vi "Untitled 1 (SubVI).vi"(0 "Byte Stream File in":refnum<file>, 1 "file open?":bool, 2 "CSV Data Headings":string, 3 "millisecond timer value in":u32, 4 "Start Logging":bool, 5 "error in (no error)":errorcluster, 6 "Log Filepath Selection":T2, 7 "adam5000:all-data-out":T3) -> (10 "appended path for log file":path, 12 "UI Element State":T1(ring), 13 "log-elapsed time":dbl format="%.2f", 14 "Byte Stream File out":refnum<file>, 15 "millisecond timer value out":u32, 16 "Logged Data String":string, 17 "Boolean":bool, 18 "Boolean 2":bool, 19 "error out":errorcluster)   [LabVIEW 2024]
uses:
  controls/thermocouple-input-cluster.ctl
  controls/analog-input-cluster.ctl
  controls/analog-output-cluster.ctl
  controls/digitial-input-cluster.ctl
  controls/digital-output-cluster.ctl
  controls/adam-5000-all-module-datas.ctl
  controls/adam-5000-all-chassis-data.ctl
  csv-file-logging/filepath-selection.ctl
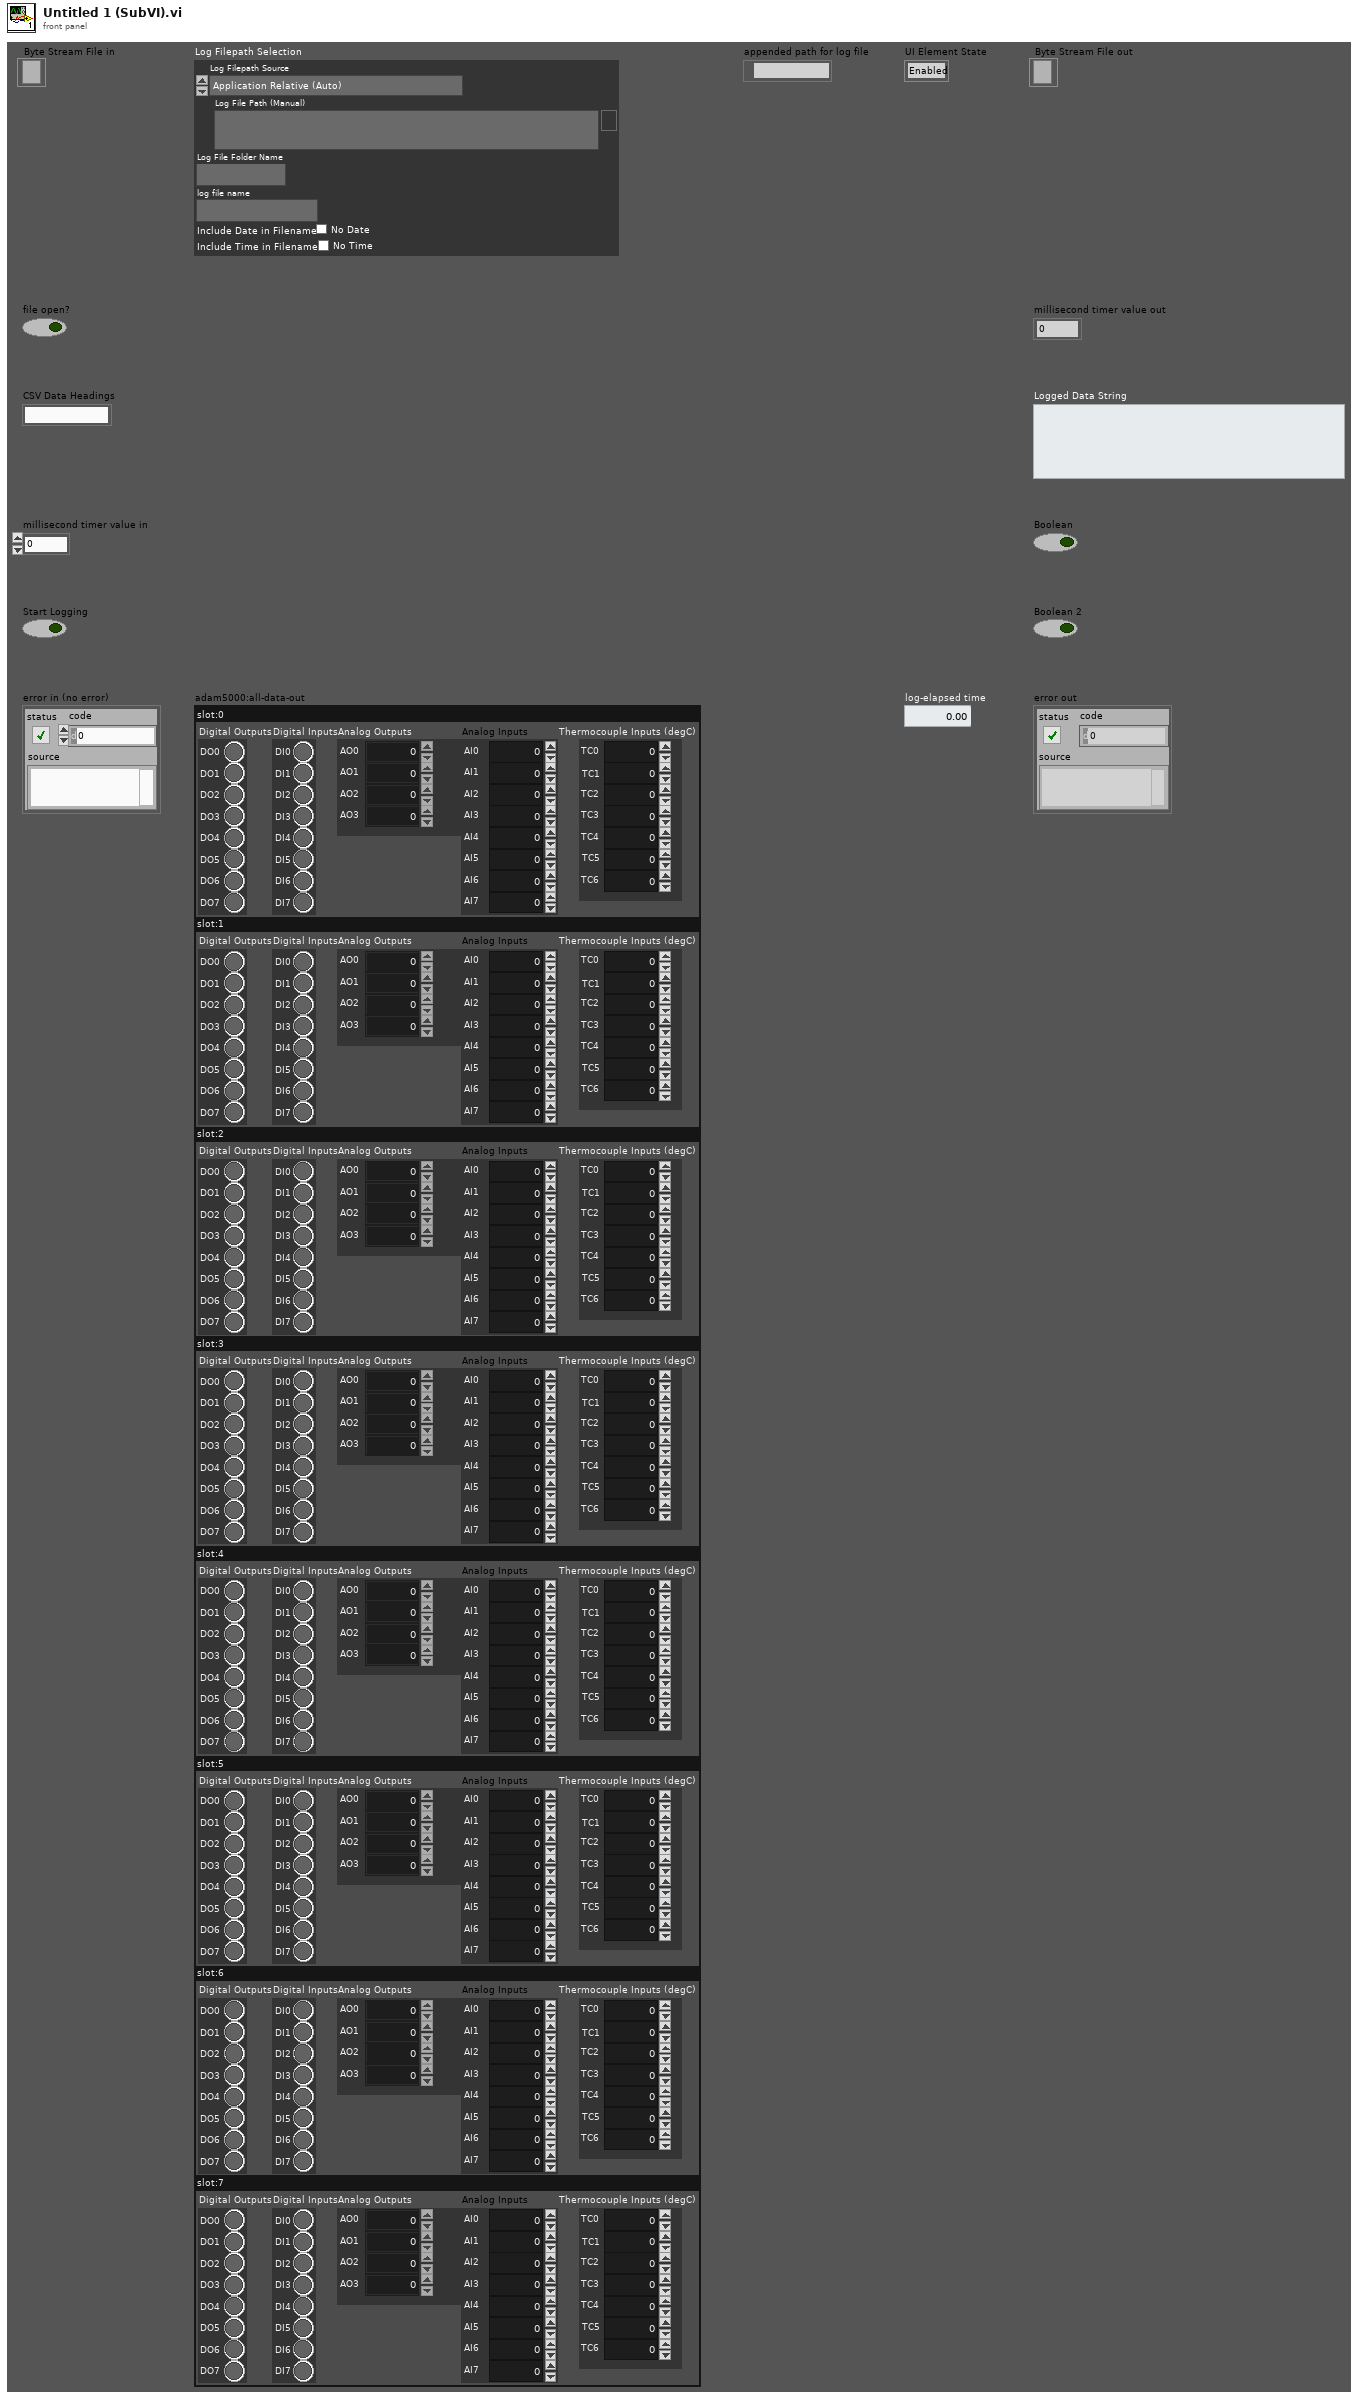
[diagram p1: front panel]
types:
  T1 = enum8{"Enabled", "Disabled", "Disabled and Grayed Out"}
  T2 = typedef "filepath-selection.ctl" = cluster{"Log Filepath Source":enum16{"Application Relative (Auto)", "VI Relative (Auto)", "Complete Path (Manual)"}, "Log File Path (Manual)":path, "Log File Folder Name":string, "log file name":string, "Include Date in Filename":bool, "Include Time in Filename":bool}
  T3 = typedef "adam-5000-all-chassis-data.ctl" = cluster{"slot:0":T4, "slot:1":T4, "slot:2":T4, "slot:3":T4, "slot:4":T4, "slot:5":T4, "slot:6":T4, "slot:7":T4}
  T4 = typedef "adam-5000-all-module-datas.ctl" = cluster{"Digital Outputs":T5, "Digital Inputs":T6, "Analog Outputs":T7, "Analog Inputs":T8, "Thermocouple Inputs (degC)":T9}
  T5 = typedef "digital-output-cluster.ctl" = cluster{"DO0":bool, "DO1":bool, "DO2":bool, "DO3":bool, "DO4":bool, "DO5":bool, "DO6":bool, "DO7":bool}
  T6 = typedef "digitial-input-cluster.ctl" = cluster{"DI0":bool, "DI1":bool, "DI2":bool, "DI3":bool, "DI4":bool, "DI5":bool, "DI6":bool, "DI7":bool}
  T7 = typedef "analog-output-cluster.ctl" = cluster{"AO0":dbl, "AO1":dbl, "AO2":dbl, "AO3":dbl}
  T8 = typedef "analog-input-cluster.ctl" = cluster{"AI0":dbl, "AI1":dbl, "AI2":dbl, "AI3":dbl, "AI4":dbl, "AI5":dbl, "AI6":dbl, "AI7":dbl}
  T9 = typedef "thermocouple-input-cluster.ctl" = cluster{"TC0":dbl, "TC1":dbl, "TC2":dbl, "TC3":dbl, "TC4":dbl, "TC5":dbl, "TC6":dbl}
  T10 = enum16{"open", "replace", "create", "open or create", "replace or create", "replace or create with confirmation"}
  T11 = cluster{"TC0":string, "TC1":string, "TC2":string, "TC3":string, "TC4":string, "TC5":string, "TC6":string}
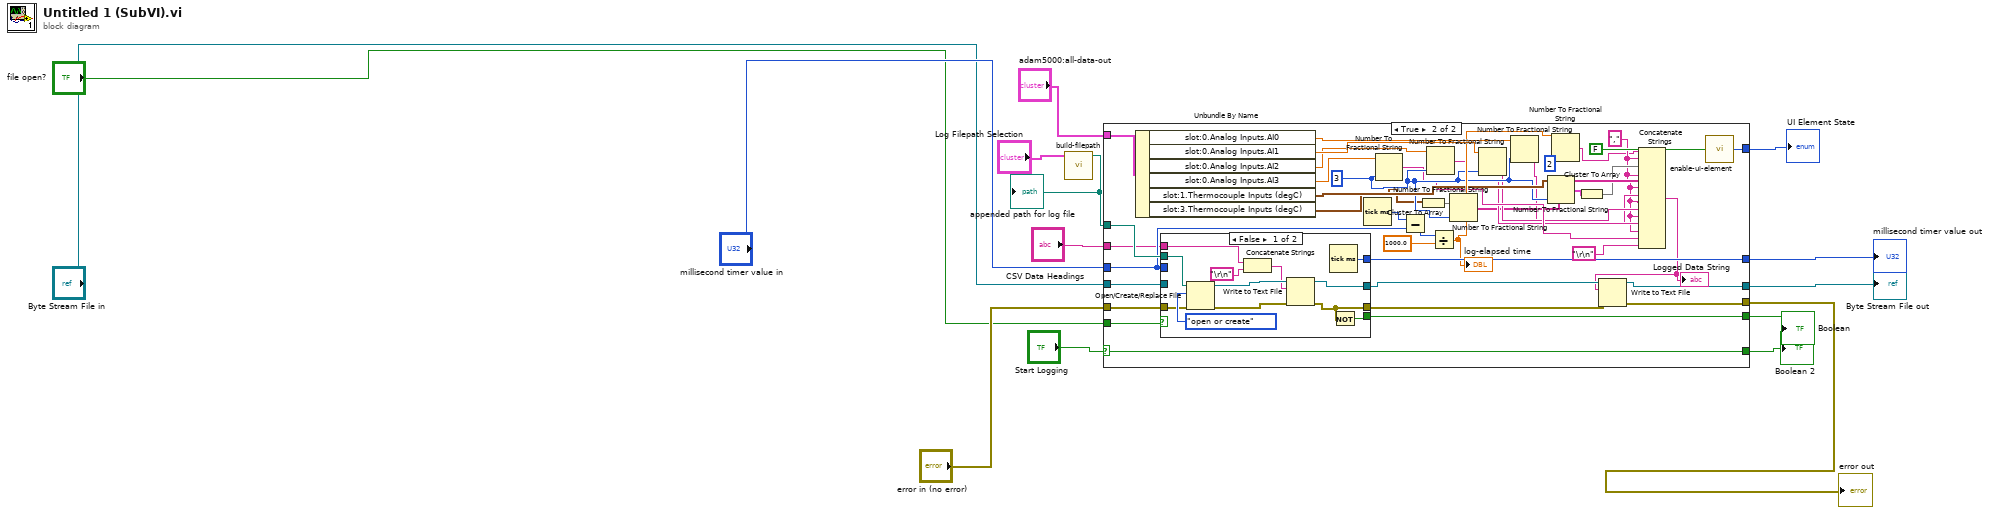
[diagram p0: block diagram]
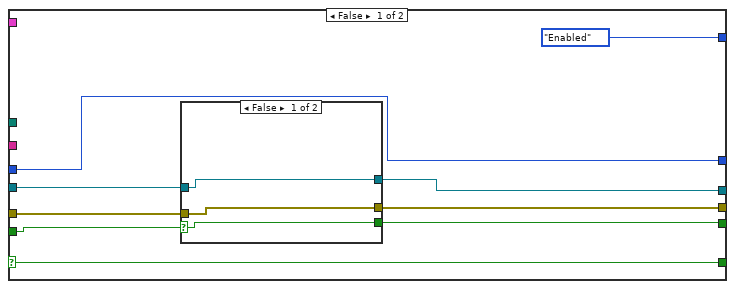
[diagram p2: hidden frame]
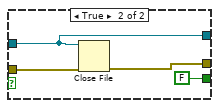
[diagram p3: hidden frame]
diagram:
  n1 = call "build-filepath.vi"("Log Filepath Selection"="Log Filepath Selection") -> ("appended path for log file"=w5:path)  [unwired: 9 in, 1 out]
  "appended path for log file" <- w5
  n2 = case shown="True" "Start Logging" {
    selector: "Start Logging" -> [w24 w68]
    tunnel: [w24 w68] -> w2
    tunnel: [T1."Enabled" ("DisabledEnum") w69] -> w3
    tunnel: w5 -> [_ w66]
    tunnel: "adam5000:all-data-out" -> [_ w71]
    tunnel: [w21 w64] -> w7
    tunnel: "file open?" -> [w22 w67]
    tunnel: "error in (no error)" -> [w19 w65]
    tunnel: [w18 w53] -> w10
    tunnel: [w17 w55] -> w11
    tunnel: "Byte Stream File in" -> [w20 w63]
    tunnel: [w16 w62] -> w13
    tunnel: "millisecond timer value in" -> [w16 w60]
    tunnel: "CSV Data Headings" -> [_ w57]
    frame False {
      n3 = case shown="False" w22 {
        selector: w22 -> [w25 _]
        tunnel: [w25 FALSE] -> w21
        tunnel: w20 -> [w27 w28]
        tunnel: w19 -> [w26 w30]
        tunnel: [w26 w29] -> w18
        tunnel: [w27 w28] -> w17
        frame False {
        }
        frame True {
          n4 = Close File(refnum=w28, error in=w30) -> (error out=w29:errorcluster)  [unwired: 1 out]
        }
      }
    }
    frame True {
      w33 = "," ("string")
      w44 = i16 3 ("precision (6)")
      n5 = Unbundle By Name(w71) -> ("slot:0.Analog Inputs.AI0"=w51:dbl, "slot:0.Analog Inputs.AI1"=w50:dbl, "slot:0.Analog Inputs.AI2"=w49:dbl, "slot:0.Analog Inputs.AI3"=w48:dbl, "slot:1.Thermocouple Inputs (degC)"=w45:T9, "slot:3.Thermocouple Inputs (degC)"=w41:T9)
      n6 = case shown="False" w67 {
        selector: w67 -> [_ w87]
        tunnel: w66 -> [w82 _]
        tunnel: w65 -> [w81 w86]
        tunnel: [w76 w86] -> w54
        tunnel: [w80 w87] -> w64
        tunnel: [w75 w84] -> w56
        tunnel: w63 -> [_ w84]
        tunnel: [w79 w85] -> w62
        tunnel: w60 -> [_ w85]
        tunnel: w57 -> [w73 _]
        frame False {
          n7 = Open/Create/Replace File(file path (use dialog)=w82, error in=w81, operation (0:open)=T10."open or create") -> (refnum out=w78:refnum<file>, error out=w77:errorcluster)  [unwired: 3 in, 1 out]
          n8 = Concatenate Strings(w73, "\r\n") -> (w72:string)
          n9 = Write to Text File(file (use dialog)=w78, text=w72, error in=w77) -> (refnum out=w75:refnum<file>, error out=w76:errorcluster)  [unwired: 1 in, 1 out]
          n10 = Tick Count (ms)() -> (millisecond timer value=w79:u32)
          n11 = Not(x=w76) -> (.not. x?=w80:bool)
        }
        frame True {
        }
      }
      n12 = Tick Count (ms)() -> (millisecond timer value=w61:u32)
      n13 = Number To Fractional String(number=w48, precision (6)=w44) -> (F-format string=w39:string)  [unwired: 2 in]
      n14 = Subtract(x=w61, y=w60) -> (x-y=w59:u32)
      n15 = Cluster To Array(cluster=w41) -> (array=w40:dbl[])
      n16 = Number To Fractional String(number=w49, precision (6)=w44) -> (F-format string=w38:string)  [unwired: 2 in]
      n17 = Divide(x=w59, y=1000.0) -> (x/y=w46:dbl)
      "log-elapsed time" <- w46
      n18 = Number To Fractional String(number=w40, precision (6)=w44) -> (F-format string=w35:string[])  [unwired: 2 in]
      n19 = Number To Fractional String(number=w50, precision (6)=w44) -> (F-format string=w37:string)  [unwired: 2 in]
      n20 = Number To Fractional String(number=w51, precision (6)=w44) -> (F-format string=w36:string)  [unwired: 2 in]
      n21 = Number To Fractional String(number=w45, precision (6)=w44) -> (F-format string=w43:T11)  [unwired: 2 in]
      n22 = Number To Fractional String(number=w46, precision (6)=i16 2) -> (F-format string=w32:string)  [unwired: 2 in]
      n23 = Cluster To Array(cluster=w43) -> (array=w34:string[])
      n24 = Concatenate Strings(w32, w33, w34, w33, w35, w33, w36, w33, w37, w33, w38, w33, w39, "\r\n") -> (w52:string)
      "Logged Data String" <- w52
      n25 = Write to Text File(file (use dialog)=w56, text=w52, error in=w54) -> (refnum out=w55:refnum<file>, error out=w53:errorcluster)  [unwired: 1 in, 1 out]
      n26 = call "enable-ui-element.vi"("Enable UI Element"=FALSE) -> ("UI Element State"=w69:T1)  [unwired: 8 in]
    }
  }
  "millisecond timer value out" <- w13
  "Byte Stream File out" <- w11
  "error out" <- w10
  "Boolean" <- w7
  "UI Element State" <- w3
  "Boolean 2" <- w2
